vi "1D_stats_labels.vi"(2 "Mode selector":T4(ring)=enum."4th Order Stats", 3 "Analysis Info Cluster":T1={"Colour"=0, "Inst type"=enum."Pitot-static tube", "Inst name"="Manometer voltage", "Symbol"="U", "Code name"="", "Extra Info"="U", "Inst Array"=enum."PWA", "Extra Titles"=[], "Extra Values"=[], "U"=0.0, "u^2"=0.0, "u^3"=0.0, "u^4"=0.0, "Skew_u"=0.0, "Kurt_u"=0.0, "Sd Error in Mean"=0.0, "% u'/U"=0.0, "X"=0.0, "Y"=0.0, "Z"=0.0, "Timescale integral Estimate"=0.0, "Sd Error in Variance"=0.0, "Calib File"=path "", "Calib Constants"=[], "Output Position"=FALSE, "Full Stats"=FALSE, "Av Sampling Rate"=0.0, "Av No of Samples"=0.0, "Total Meas Time (s)"=0.0, "ADAM Ch Name"="", "Max value"=0.0, "Min value"=0.0} {"Sd Error in Variance" format="%.2f"; "Skew_u" format="%.2f"; "% u'/U" format="%.2f"; "Sd Error in Mean" format="%.2f"; "Kurt_u" format="%.2f"; "u^4" format="%.2f"; "u^3" format="%.2f"; "U" format="%.2f"; "u^2" format="%.2f"}) -> (0 "Output":string[](array[string]))   [LabVIEW 2016]
uses:
  Controls/Analysis_info_cluster.ctl
  Controls/Inst_type.ctl
  Controls/Instrument_Array.ctl
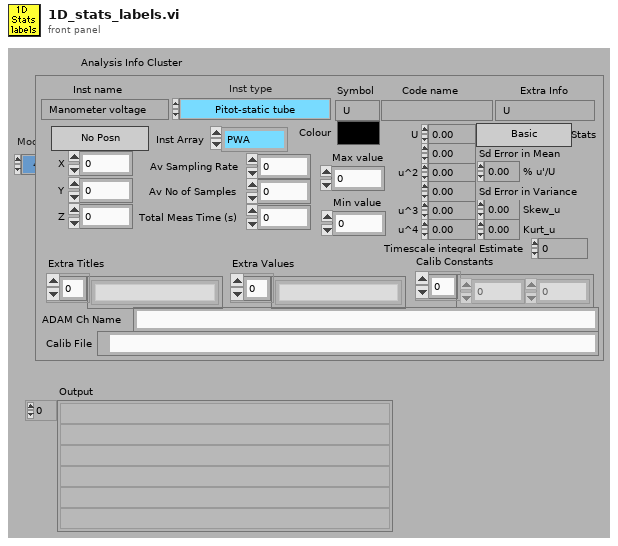
[diagram p1: front panel]
types:
  T1 = typedef "Analysis_info_cluster.ctl" = cluster{"Colour":u32, "Inst type":T2, "Inst name":string, "Symbol":string, "Code name":string, "Extra Info":string, "Inst Array":T3, "Extra Titles":string[], "Extra Values":string[], "U":dbl, "u^2":dbl, "u^3":dbl, "u^4":dbl, "Skew_u":dbl, "Kurt_u":dbl, "Sd Error in Mean":dbl, "% u'/U":dbl, "X":dbl, "Y":dbl, "Z":dbl, "Timescale integral Estimate":dbl, "Sd Error in Variance":dbl, "Calib File":path, "Calib Constants":dbl[], "Output Position":bool, "Full Stats":bool, "Av Sampling Rate":dbl, "Av No of Samples":dbl, "Total Meas Time (s)":dbl, "ADAM Ch Name":string, "Max value":dbl, "Min value":dbl}
  T2 = typedef "Inst_type.ctl" = enum16{"Propeller anemometer", "Raw voltage", "Pressure Transducer", "Pitot-static tube", "Preston tube", "Hot wire", "Cross wire 1", "Cross wire 2", "Generic Linear", "Generic Polynomial", "Generic BackPoly", "Fast FID", "Thermocouple", "Cold wire", "Pulsed Wire", "LDA Vel", "LDA Tran time", "LDA Arr time", "Microphone"}
  T3 = typedef "Instrument_Array.ctl" = enum16{"PWA", "LDA", "Analogue"}
  T4 = enum16{"Mean only", "2nd Order Stats", "4th Order Stats"}
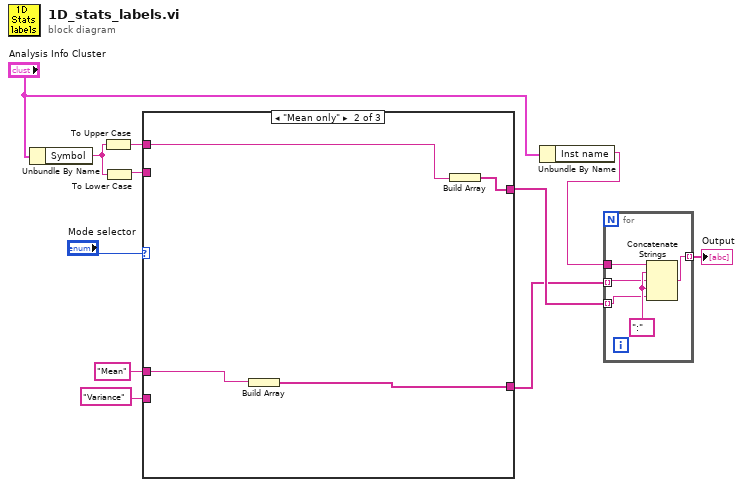
[diagram p0: block diagram]
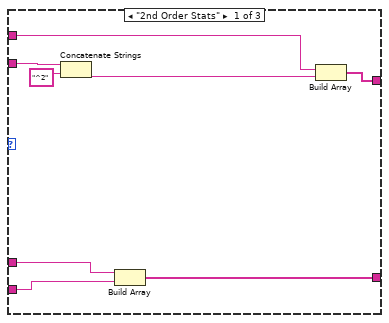
[diagram p2: hidden frame]
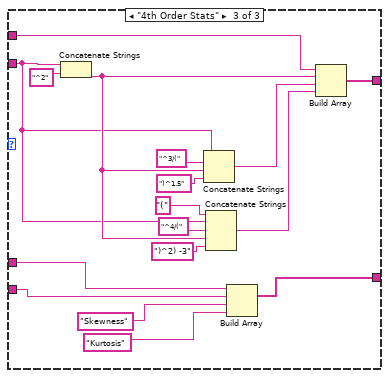
[diagram p3: hidden frame]
diagram:
  n1 = Unbundle By Name("Analysis Info Cluster") -> ("Symbol"=w5:string)
  n2 = To Upper Case(1:w5) -> (0:w10:string)
  n3 = To Lower Case(string=w5) -> (all lower case string=w9:string)
  n4 = case shown="\"Mean only\"" "Mode selector" {
    tunnel: w10 -> [w19 w23 w40]
    tunnel: w9 -> [w16 _ w32]
    tunnel: [w17 w22 w30] -> w3
    tunnel: "Mean" -> [w14 w21 w26]
    tunnel: "Variance" -> [w13 _ w27]
    tunnel: [w12 w20 w25] -> w2
    frame "2nd Order Stats" {
      n5 = Concatenate Strings(w16, "^2") -> (w15:string)
      n6 = Build Array(w14, w13) -> (w12:string[])
      n7 = Build Array(w19, w15) -> (w17:string[])
    }
    frame "Mean only" {
      n8 = Build Array(w21) -> (w20:string[])
      n9 = Build Array(w23) -> (w22:string[])
    }
    frame "4th Order Stats" {
      n10 = Concatenate Strings(w32, "^2") -> (w33:string)
      n11 = Concatenate Strings(w32, "^3/(", w33, ")^1.5") -> (w36:string)
      n12 = Concatenate Strings("(", w32, "^4/(", w33, ")^2) -3") -> (w31:string)
      n13 = Build Array(w26, w27, "Skewness", "Kurtosis") -> (w25:string[])
      n14 = Build Array(w40, w33, w36, w31) -> (w30:string[])
    }
  }
  n15 = Unbundle By Name("Analysis Info Cluster") -> ("Inst name"=w1:string)
  n16 = for {
    tunnel: [w45] -> w6 mode=indexing
    tunnel: w1 -> [w44]
    tunnel: w2 -> [w42] mode=indexing
    tunnel: w3 -> [w41] mode=indexing
    w43 = ":" ("Substring")
    n17 = Concatenate Strings(w44, w43, w42, w43, w41) -> (w45:string)
  }
  "Output" <- w6
